vi "Model - DeInit.vi"(8 "error in (no error)":errorcluster, 11 "View Model":T1) -> (0 "error out":errorcluster)   [LabVIEW 2017]
doc: "Deinitialize View Model user events and DVRs"
uses:
  Controls/View Model.ctl
  Error Handler/Controls/Error Model.ctl
  Error Handler/Controls/Error EventData.ctl
  Error Handler/Controls/Error Type.ctl
  Elevator Controller/Controls/Elevator Model.ctl
  Elevator Controller/Controls/Elevator Overhead.ctl
  Elevator Controller/Controls/Elevator States.ctl
  Elevator Controller/Controls/Elevator Location.ctl
  Elevator Controller/Controls/Elevator Command Event.ctl
  Elevator Controller/Controls/Elevator Commands.ctl
  Configuration/Controls/Configuration Model.ctl
  Configuration/Controls/Configuration Data.ctl
  Controls/Shared Model.ctl
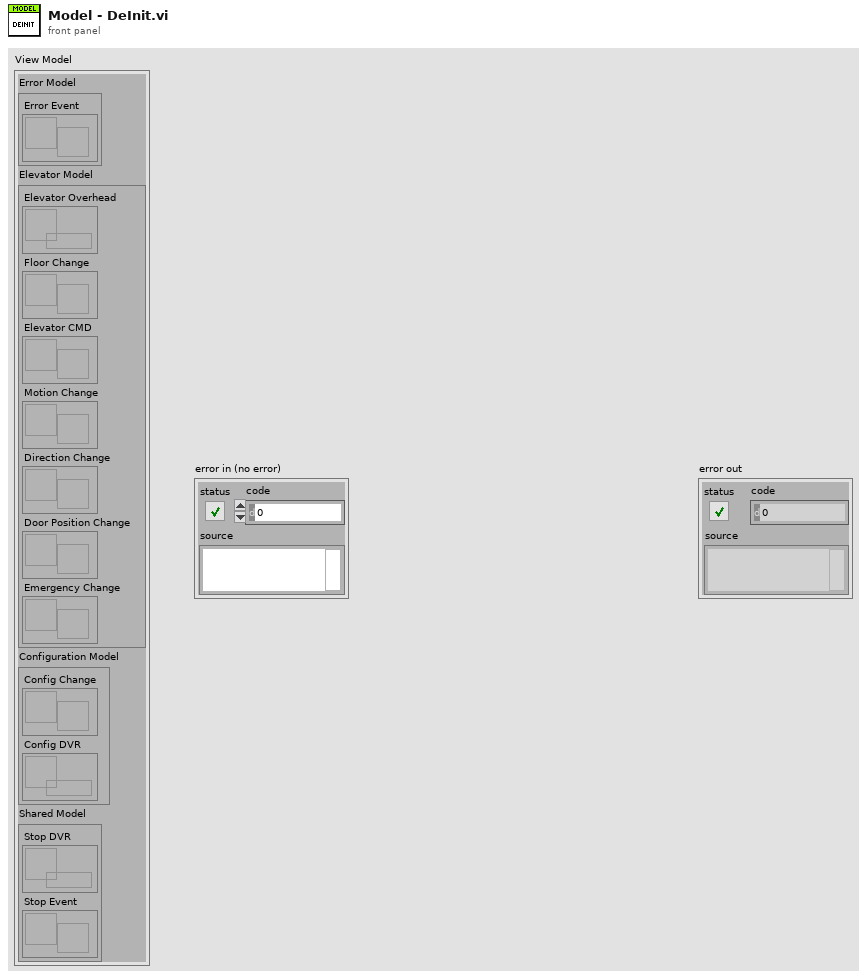
[diagram p1: front panel]
types:
  T1 = typedef "View Model.ctl" = cluster{"Error Model":T2, "Elevator Model":T3, "Configuration Model":T4, "Shared Model":T5}
  T2 = typedef "Error Model.ctl" = cluster{"Error Event":refnum<user-event>}
  T3 = typedef "Elevator Model.ctl" = cluster{"Elevator Overhead":refnum<data-value>, "Floor Change":refnum<user-event>, "Elevator CMD":refnum<user-event>, "Motion Change":refnum<user-event>, "Direction Change":refnum<user-event>, "Door Position Change":refnum<user-event>, "Emergency Change":refnum<user-event>}
  T4 = typedef "Configuration Model.ctl" = cluster{"Config Change":refnum<user-event>, "Config DVR":refnum<data-value>}
  T5 = typedef "Shared Model.ctl" = cluster{"Stop DVR":refnum<data-value>, "Stop Event":refnum<user-event>}
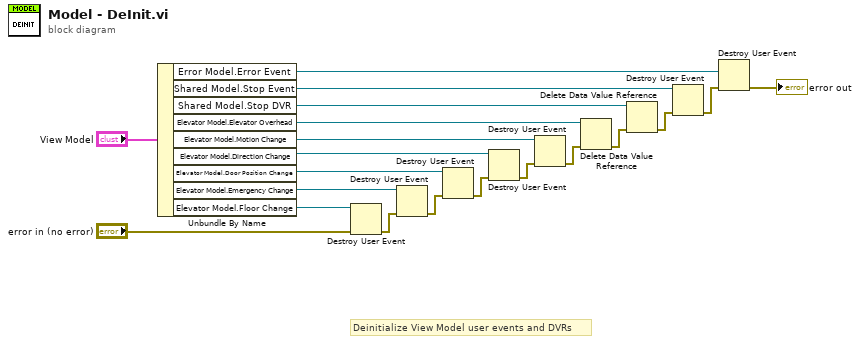
[diagram p0: block diagram]
diagram:
  # "Deinitialize View Model user events and DVRs"
  n1 = Unbundle By Name("View Model") -> ("Error Model.Error Event"=w19:refnum<user-event>, "Shared Model.Stop Event"=w7:refnum<user-event>, "Shared Model.Stop DVR"=w6:refnum<data-value>, "Elevator Model.Elevator Overhead"=w5:refnum<data-value>, "Elevator Model.Motion Change"=w4:refnum<user-event>, "Elevator Model.Direction Change"=w3:refnum<user-event>, "Elevator Model.Door Position Change"=w2:refnum<user-event>, "Elevator Model.Emergency Change"=w1:refnum<user-event>, "Elevator Model.Floor Change"=w18:refnum<user-event>)
  n2 = Destroy User Event(user event=w18, error in="error in (no error)") -> (error out=w16:errorcluster)
  n3 = Destroy User Event(user event=w1, error in=w16) -> (error out=w15:errorcluster)
  n4 = Destroy User Event(user event=w2, error in=w15) -> (error out=w14:errorcluster)
  n5 = Destroy User Event(user event=w3, error in=w14) -> (error out=w13:errorcluster)
  n6 = Destroy User Event(user event=w4, error in=w13) -> (error out=w12:errorcluster)
  n7 = Delete Data Value Reference(data value reference=w5, error in=w12) -> (error out=w11:errorcluster)  [unwired: 1 out]
  n8 = Delete Data Value Reference(data value reference=w6, error in=w11) -> (error out=w10:errorcluster)  [unwired: 1 out]
  n9 = Destroy User Event(user event=w7, error in=w10) -> (error out=w9:errorcluster)
  n10 = Destroy User Event(user event=w19, error in=w9) -> (error out=→"error out":errorcluster)
